vi "XY Plotter Main.vi"() -> ()   [LabVIEW 2024]
uses:
  Msg.ctl
  Msg_Type.ctl
  <vilib>/DAQmx/read.llb/DAQmx Read (Analog 2D DBL NChan NSamp).vi
  <vilib>/DAQmx/create/channels.llb/DAQmx Create Channel (AI-Voltage-Basic).vi
  <vilib>/DAQmx/configure/timing.llb/DAQmx Timing (Sample Clock).vi
  <vilib>/DAQmx/miscellaneous.llb/DAQmx Fill In Error Info.vi
  <vilib>/Utility/file.llb/Write Delimited Spreadsheet (DBL).vi
  <vilib>/Utility/file.llb/Read Delimited Spreadsheet (DBL).vi
panel:
  out "error out":errorcluster
  out "all rows":dbl[][](array[numeric])
  in  "Load":bool
  in  "Pen":bool
  in  "Save Button":bool
  in  "Path":path
  out "XY Graph":cluster{dbl[], "Trace y":dbl[]}(graph)
  in  "Physical Device channels":tag
  in  "Sample hertz":dbl
  in  "Exit":bool
  in  "Clear Graph":bool
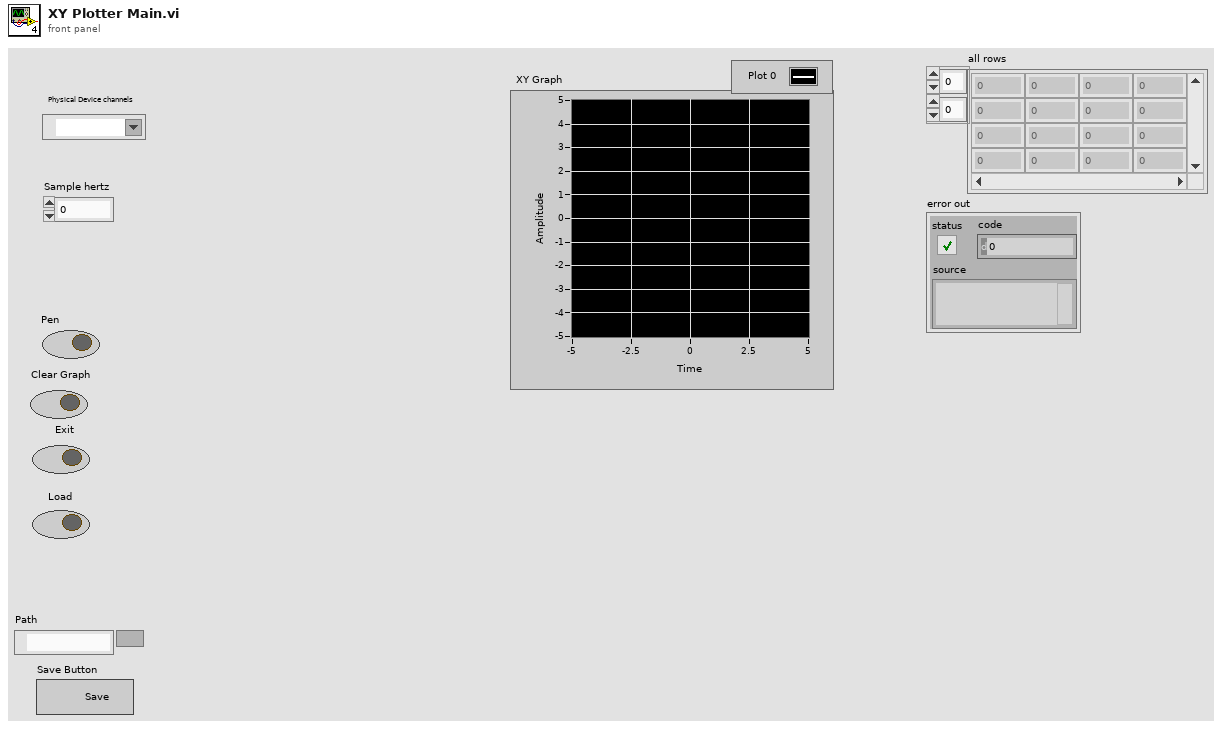
[diagram p1: front panel]
types:
  T1 = typedef "Msg.ctl" = cluster{"Type":T2, "Sample Rate(HZ)":dbl, "X-Array":dbl[], "Y-Array":dbl[]}
  T2 = typedef "Msg_Type.ctl" = enum16{"", "Pen", "Start", "Stop", "CLear", "Save", "load", "Exit", "UpdateSampleRate", "NewData"}
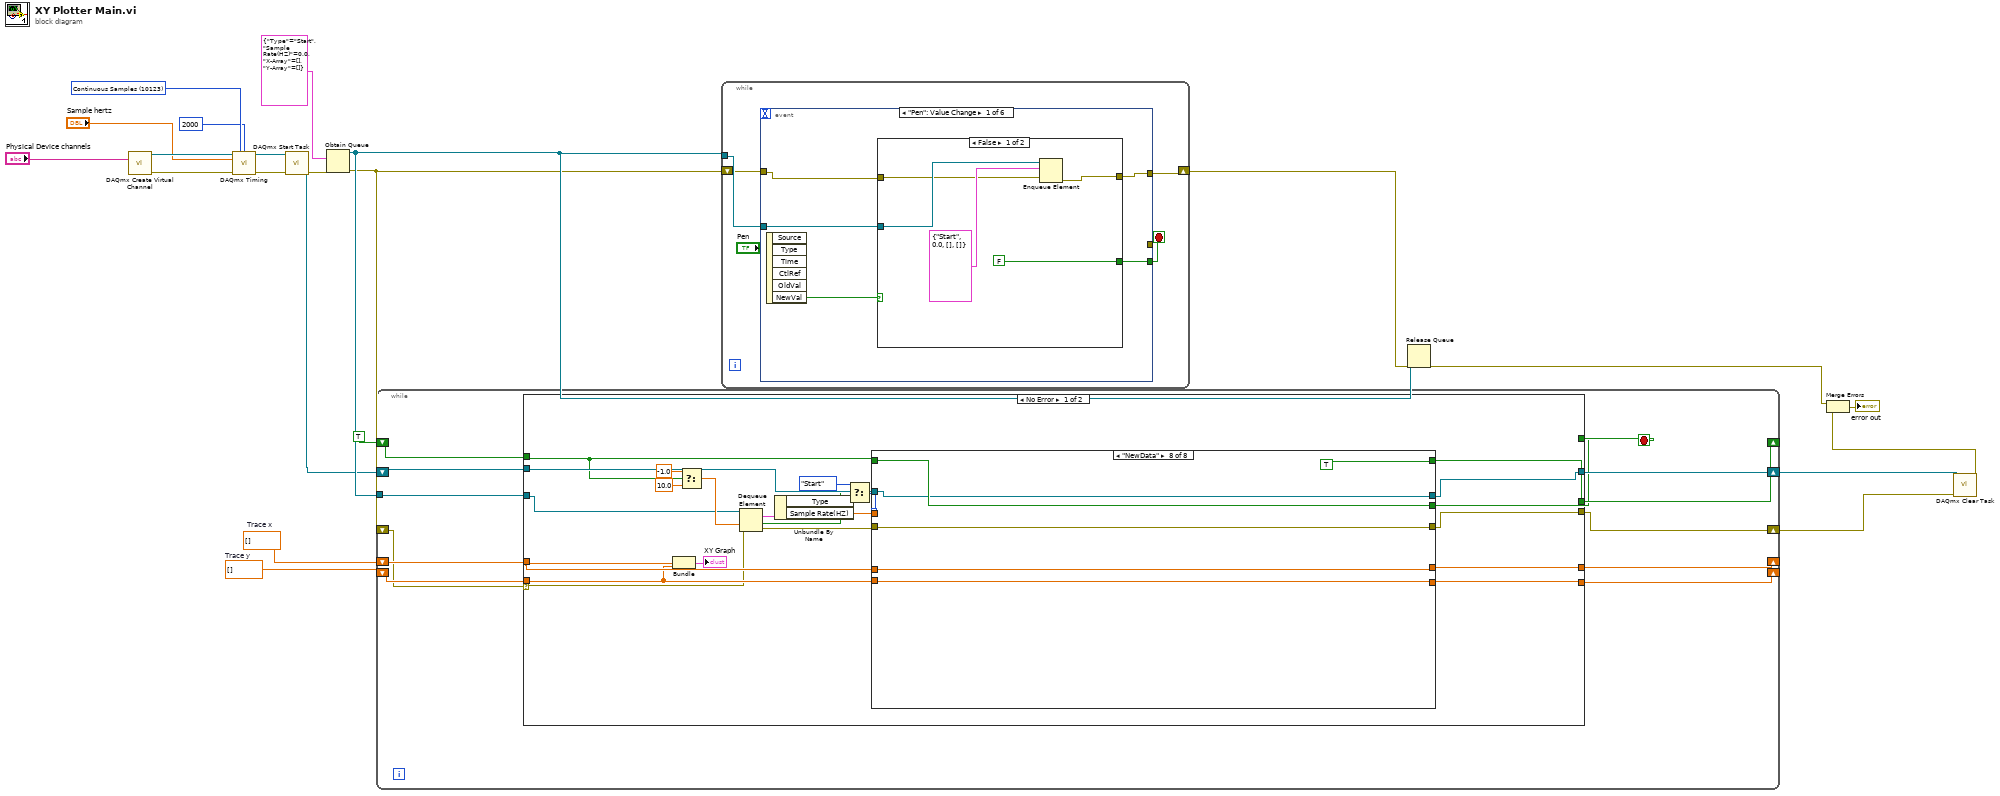
[diagram p0: block diagram]
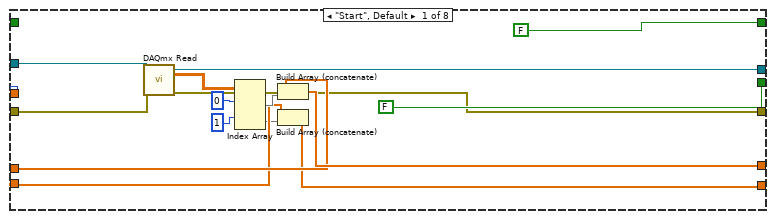
[diagram p2: hidden frame]
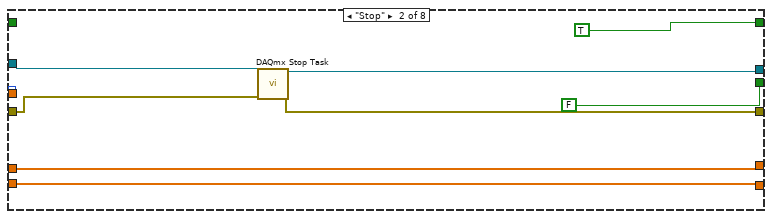
[diagram p3: hidden frame]
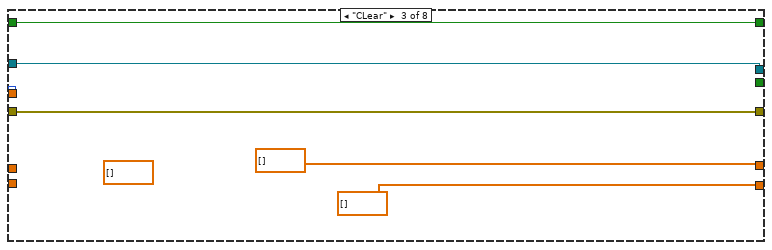
[diagram p4: hidden frame]
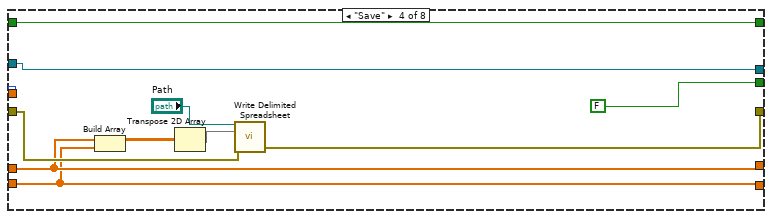
[diagram p5: hidden frame]
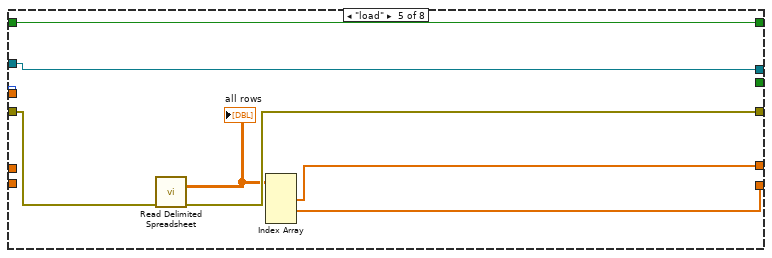
[diagram p6: hidden frame]
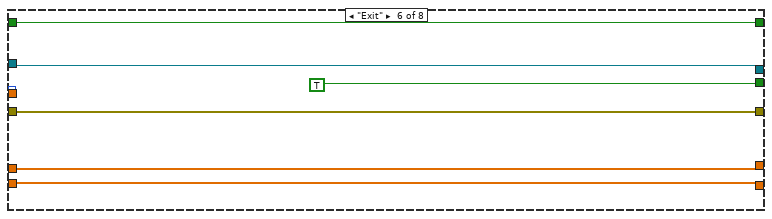
[diagram p7: hidden frame]
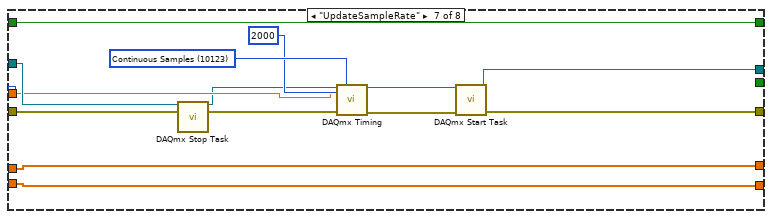
[diagram p8: hidden frame]
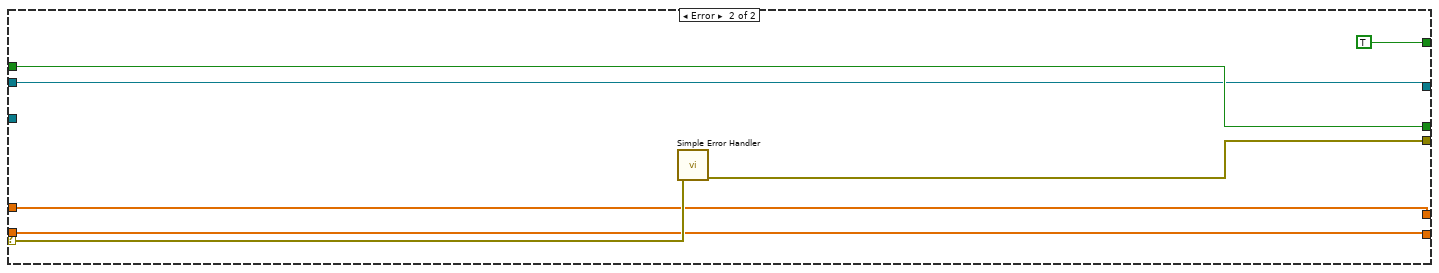
[diagram p9: hidden frame]
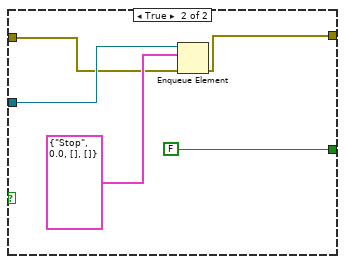
[diagram p10: hidden frame]
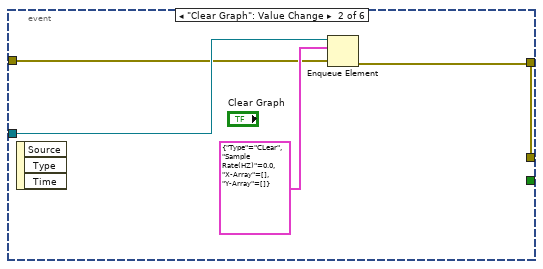
[diagram p11: hidden frame]
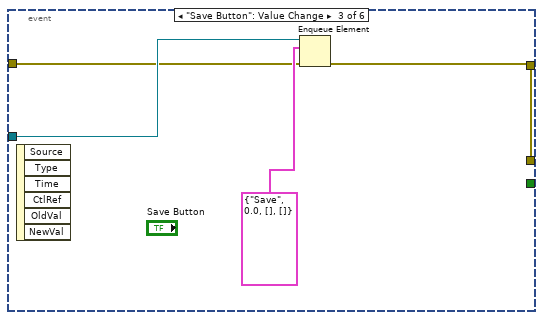
[diagram p12: hidden frame]
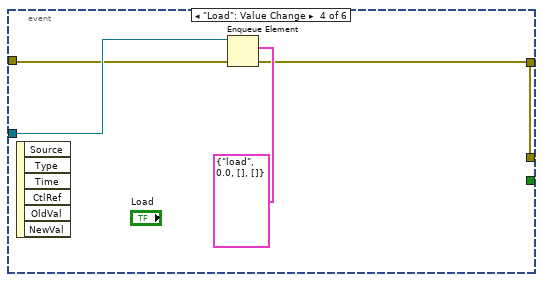
[diagram p13: hidden frame]
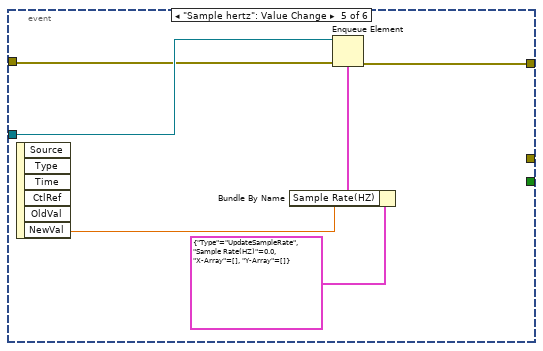
[diagram p14: hidden frame]
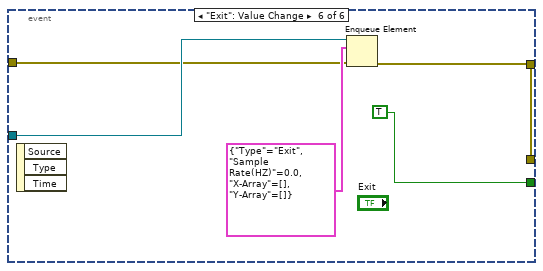
[diagram p15: hidden frame]
diagram:
  w9 = dbl[] []  # Trace x
  w16 = 10123 items=["Finite Samples"=10178, "Continuous Samples"=10123, "Hardware Timed Single Point"=12522] ("sample mode")
  w20 = dbl[] []  # Trace y
  n1 = call-poly <vilib>:"DAQmx Create Virtual Channel.vi"("physical channels"="Physical Device channels") -> ("task out"=w18:refnum<k21>, "error out"=w13:errorcluster)  [unwired: 13 in]
  n2 = call-poly <vilib>:"DAQmx Timing.vi"("task/channels in"=w18, "sample mode"=w16, "samples per channel"=2000, "rate"="Sample hertz", "error in"=w13) -> ("task out"=w14:refnum<k21>, "error out"=w12:errorcluster)  [unwired: 9 in]
  n3 = call <vilib>:"DAQmx Start Task.vi"("task/channels in"=w14, "error in"=w12) -> ("task out"=w10:refnum<k21>, "error out"=w7:errorcluster)  [unwired: 12 in]
  n4 = Obtain Queue(element data type=T1 {"Type"=enum."Start", "Sample Rate(HZ)"=0.0, "X-Array"=[], "Y-Array"=[]} ("Cluster"), error in (no error)=w7) -> (queue out=w22:refnum<queue>, error out=w2:errorcluster)  [unwired: 3 in, 1 out]
  n5 = while {
    tunnel: w22 -> [w34]
    shift-right: [w27] -> _
    shift-left: TRUE -> [w23]
    shift-right: [w33] -> _
    shift-left: w20 -> [w31]
    shift-right: [w30] -> _
    shift-left: w9 -> [w32]
    shift-right: [w26] -> w6
    shift-left: w10 -> [w29]
    shift-right: [w24] -> w1
    shift-left: w2 -> [w25]
    stop <- w28 stop-if-true
    n6 = case shown="No Error" w25 {
      selector: w25 -> [w39 w132]
      tunnel: w34 -> [w37 _]
      tunnel: [w55 w128] -> w33
      tunnel: w32 -> [w54 w129]
      tunnel: w31 -> [w53 w128]
      tunnel: [w51 w129] -> w30
      tunnel: w29 -> [w50 w131]
      tunnel: w23 -> [w38 w133]
      tunnel: [w44 TRUE] -> w28
      tunnel: [w42 w133] -> w27
      tunnel: [w36 w131] -> w26
      tunnel: [w35 w130] -> w24
      frame No Error {
        n7 = Bundle("Trace x"=w54, "Trace y"=w53) -> (→"XY Graph":cluster{"Trace x":dbl[], "Trace y":dbl[]})  [unwired: 1 in]
        n8 = Select(t=-1.0, s=w38, f=10.0) -> (s? t:f=w47:dbl)
        n9 = Dequeue Element(queue=w37, timeout in ms (-1)=w47, error in (no error)=w39) -> (element=w57:T1, timed out?=w46:bool, error out=w56:errorcluster)  [unwired: 1 out]
        n10 = Unbundle By Name(w57) -> ("Type"=w43:T2, "Sample Rate(HZ)"=w40:dbl)
        n11 = Select(t=Msg_Type."Start", s=w46, f=w43) -> (s? t:f=w45:T2)
        n12 = case shown="\"NewData\"" w45 {
          tunnel: [FALSE TRUE w81 w88 w96 w107 w114 TRUE] -> w42
          tunnel: w54 -> [w66 w79 _ w92 _ w104 w119 w121]
          tunnel: w53 -> [w64 w80 _ w91 _ w106 w120 w125]
          tunnel: w38 -> [_ _ w81 w88 w96 w107 w114 w123]
          tunnel: [w67 w79 dbl[] [] w92 w98 w104 w119 w121] -> w51
          tunnel: [w62 w80 dbl[] [] ("Trace y") w91 w97 w106 w120 w125] -> w55
          tunnel: w56 -> [w59 w77 w85 w93 w102 w105 w109 w124]
          tunnel: [w58 w76 w85 w86 w101 w105 w109 w124] -> w35
          tunnel: [FALSE FALSE _ FALSE _ TRUE _ w123] -> w44
          tunnel: w50 -> [w60 w78 w84 w90 w100 w103 w115 w122]
          tunnel: [w72 w75 w84 w90 w100 w103 w113 w122] -> w36
          tunnel: w40 -> [_ _ _ _ _ _ w112 _]
          frame "Start", Default {
            n13 = call-poly <vilib>:"DAQmx Read.vi"("task/channels in"=w60, "error in"=w59) -> ("task out"=w72:refnum<k21>, "data"=w71:dbl[][], "error out"=w58:errorcluster)  [unwired: 11 in]
            n14 = Index Array(array=w71, index (row) #1=0 ("index (row)"), index (row) #2=1 ("index (row)")) -> (element #1=w65:dbl[], element #2=w63:dbl[])  [unwired: 2 in]
            n15 = Build Array (concatenate)(w66, w65) -> (w67:dbl[])
            n16 = Build Array (concatenate)(w64, w63) -> (w62:dbl[])
          }
          frame "Stop" {
            n17 = call <vilib>:"DAQmx Stop Task.vi"("task/channels in"=w78, "error in"=w77) -> ("task out"=w75:refnum<k21>, "error out"=w76:errorcluster)  [unwired: 12 in]
          }
          frame "CLear" {
            (unwired) dbl[] []
          }
          frame "Save" {
            n18 = Build Array(w92, w91) -> (w95:dbl[][])
            n19 = Transpose 2D Array(2D array=w95) -> (transposed array=w94:dbl[][])
            n20 = call-poly <vilib>:"Write Delimited Spreadsheet.vi"("file path (dialog if empty)"="Path", "2D data"=w94, "error in (no error)"=w93) -> ("error out"=w86:errorcluster)  [unwired: 11 in, 1 out]
          }
          frame "load" {
            n21 = call-poly <vilib>:"Read Delimited Spreadsheet.vi"("error in (no error)"=w102) -> ("all rows"=w99:dbl[][], "error out"=w101:errorcluster)  [unwired: 9 in, 4 out]
            "all rows" <- w99
            n22 = Index Array(array=w99) -> (element #1=w98:dbl[], element #2=w97:dbl[])  [unwired: 4 in]
          }
          frame "Exit" {
          }
          frame "UpdateSampleRate" {
            w117 = 10123 items=["Finite Samples"=10178, "Continuous Samples"=10123, "Hardware Timed Single Point"=12522] ("sample mode")
            n23 = call <vilib>:"DAQmx Stop Task.vi"("task/channels in"=w115) -> ("task out"=w111:refnum<k21>)  [unwired: 13 in, 1 out]
            n24 = call-poly <vilib>:"DAQmx Timing.vi"("task/channels in"=w111, "sample mode"=w117, "samples per channel"=2000, "rate"=w112) -> ("task out"=w118:refnum<k21>, "error out"=w110:errorcluster)  [unwired: 10 in]
            n25 = call <vilib>:"DAQmx Start Task.vi"("task/channels in"=w118, "error in"=w110) -> ("task out"=w113:refnum<k21>)  [unwired: 12 in, 1 out]
          }
          frame "NewData" {
          }
        }
      }
      frame Error {
        n26 = call <vilib>:"Simple Error Handler.vi"("error in (no error)"=w132) -> ("error out"=w130:errorcluster)  [unwired: 4 in, 4 out]
      }
    }
  }
  n27 = while {
    tunnel: w22 -> [w137]
    shift-right: [w134] -> w8
    shift-left: w2 -> [w135]
    stop <- w136 stop-if-true
    n28 = event shown="[0] \"Pen\": Value Change" {
      selector: _ -> [_ _ _ _ _ _]
      dyn-events: _ -> [_ _ _ _ _ _]
      timeout: _ -> [_ _ _ _ _ _]
      tunnel: w137 -> [w141 w156 w160 w164 w170 w175]
      tunnel: [w140 _ _ _ _ TRUE] -> w136
      tunnel: w135 -> [w139 w154 w158 w162 w166 w172]
      tunnel: [_ w153 w157 w161 _ w171] -> _
      tunnel: [w138 _ _ _ w165 _] -> w134
      event "Pen": Value Change {
        n29 = event-data() -> ("NewVal"=w142:bool)  [unwired: 1 in, 5 out]
        n30 = case shown="False" w142 {
          tunnel: w141 -> [w147 w152]
          tunnel: [FALSE FALSE] -> w140
          tunnel: w139 -> [w144 w149]
          tunnel: [w143 w148] -> w138
          frame False {
            n31 = Enqueue Element(queue=w147, element=T1 {"Type"=enum."Start", "Sample Rate(HZ)"=0.0, "X-Array"=[], "Y-Array"=[]} ("Cluster"), error in (no error)=w144) -> (error out=w143:errorcluster)  [unwired: 1 in, 2 out]
          }
          frame True {
            n32 = Enqueue Element(queue=w152, element=T1 {"Type"=enum."Stop", "Sample Rate(HZ)"=0.0, "X-Array"=[], "Y-Array"=[]} ("Cluster"), error in (no error)=w149) -> (error out=w148:errorcluster)  [unwired: 1 in, 2 out]
          }
        }
      }
      event "Clear Graph": Value Change {
        n33 = event-data() -> ()  [unwired: 1 in, 3 out]
        n34 = Enqueue Element(queue=w156, element=T1 {"Type"=enum."CLear", "Sample Rate(HZ)"=0.0, "X-Array"=[], "Y-Array"=[]} ("Cluster"), error in (no error)=w154) -> (error out=w153:errorcluster)  [unwired: 1 in, 2 out]
      }
      event "Save Button": Value Change {
        n35 = event-data() -> ()  [unwired: 1 in, 6 out]
        n36 = Enqueue Element(queue=w160, element=T1 {"Type"=enum."Save", "Sample Rate(HZ)"=0.0, "X-Array"=[], "Y-Array"=[]} ("Cluster"), error in (no error)=w158) -> (error out=w157:errorcluster)  [unwired: 1 in, 2 out]
      }
      event "Load": Value Change {
        n37 = event-data() -> ()  [unwired: 1 in, 6 out]
        n38 = Enqueue Element(queue=w164, element=T1 {"Type"=enum."load", "Sample Rate(HZ)"=0.0, "X-Array"=[], "Y-Array"=[]} ("Cluster"), error in (no error)=w162) -> (error out=w161:errorcluster)  [unwired: 1 in, 2 out]
      }
      event "Sample hertz": Value Change {
        n39 = event-data() -> ("NewVal"=w169:dbl)  [unwired: 1 in, 5 out]
        n40 = Bundle By Name(cluster=T1 {"Type"=enum."UpdateSampleRate", "Sample Rate(HZ)"=0.0, "X-Array"=[], "Y-Array"=[]} ("Cluster"), "Sample Rate(HZ)"=w169) -> (w167:T1)
        n41 = Enqueue Element(queue=w170, element=w167, error in (no error)=w166) -> (error out=w165:errorcluster)  [unwired: 1 in, 2 out]
      }
      event "Exit": Value Change {
        n42 = event-data() -> ()  [unwired: 1 in, 3 out]
        n43 = Enqueue Element(queue=w175, element=T1 {"Type"=enum."Exit", "Sample Rate(HZ)"=0.0, "X-Array"=[], "Y-Array"=[]} ("Cluster"), error in (no error)=w172) -> (error out=w171:errorcluster)  [unwired: 1 in, 2 out]
      }
    }
  }
  n44 = Release Queue(queue=w22, error in (no error)=w8) -> (error out=w4:errorcluster)  [unwired: 1 in, 2 out]
  n45 = call <vilib>:"DAQmx Clear Task.vi"("task in"=w6, "error in"=w1) -> ("error out"=w5:errorcluster)  [unwired: 13 in]
  n46 = Merge Errors(w4, w5) -> (→"error out":errorcluster)
